vi "NIDCPower_channel_ganging - commit.vi"(8 "error in (no error)":errorcluster, 11 "Ganged Session In":T1) -> (0 "error out":errorcluster, 3 "Ganged Session Out":T1)   [LabVIEW 2021]
uses:
  ctl/NIDCPower_channel_ganging - ctl - ganged session.ctl
  ctl/NIDCPower_channel_ganging - ctl - ganged config.ctl
  ctl/NIDCPower_channel_ganging - ctl - channel mode.ctl
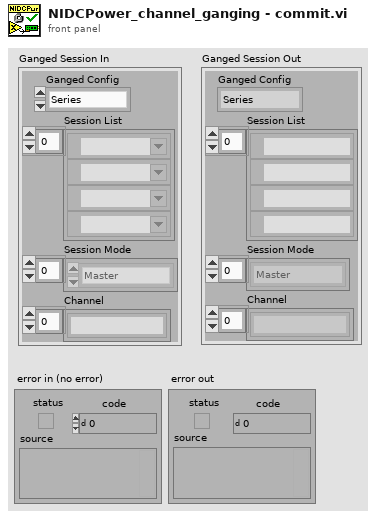
[diagram p1: front panel]
types:
  T1 = typedef "NIDCPower_channel_ganging - ctl - ganged session.ctl" = cluster{"Ganged Config":T2, "Session List":refnum<k15>[], "Session Mode":T3[], "Channel":string[]}
  T2 = typedef "NIDCPower_channel_ganging - ctl - ganged config.ctl" = enum32{"Series", "Parallel", "Manual"}
  T3 = typedef "NIDCPower_channel_ganging - ctl - channel mode.ctl" = enum32{"Master", "Slave", "Slave - Inverted"}
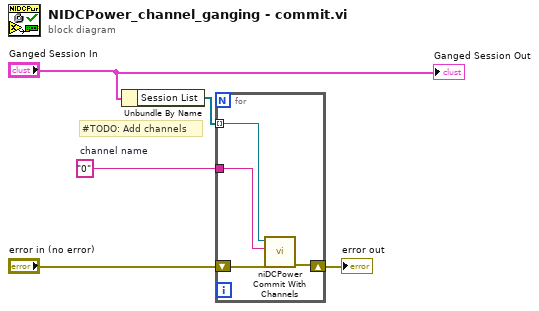
[diagram p0: block diagram]
diagram:
  w1 = "0"  # channel name
  # "#TODO: Add channels"
  n1 = Unbundle By Name("Ganged Session In") -> ("Session List"=w2:refnum<k15>[])
  n2 = for {
    shift-right: [w9] -> w4
    shift-left: "error in (no error)" -> [w8]
    tunnel: w2 -> [w7] mode=indexing
    tunnel: w1 -> [w6]
    n3 = call <instrlib>:"niDCPower Commit With Channels.vi"("error in (no error)"=w8, "channel name"=w6, "instrument handle"=w7) -> ("error out"=w9:errorcluster)  [unwired: 7 in, 1 out]
  }
  "error out" <- w4
  "Ganged Session Out" <- "Ganged Session In"
